vi "Inner Loop Control Select.vi"(8 "Inner Loop Gain Multiplier":dbl=1.0, 10 "Controller - User Input":T2={"Num Inner Loop"=[-11.0745, 19.702, -8.7598], "Den Inner Loop"=[1.0, -1.49756, 0.49756], "Inner Loop Gain"=1.0, "IMU_sample_rate"=0, "Num Outer Loop"=[0.1636, -0.16289, 0.0], "Den Outer Loop"=[1.0, -0.6326, 0.0], "Outer Loop Gain"=1.0, "Outer Loop sample rate"=20.0}, 11 "Controller Select":T1(ring)=enum."100hz/100hz" caption="Enum") -> (0 "Inner Loop Controller":T3, 4 "Outer Loop sample rate out":dbl)   [LabVIEW 2014]
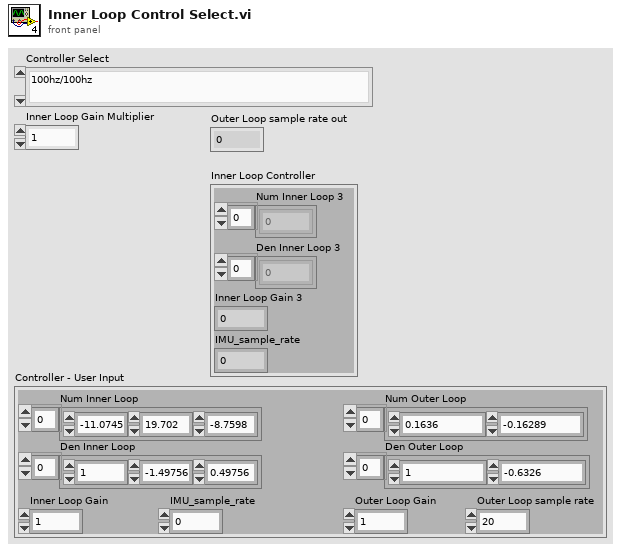
[diagram p1: front panel]
types:
  T1 = enum16{"100hz/50hz", "100hz/100hz", "200hz/200hz", "200hz/20hz", "User Defined"}
  T2 = cluster{"Num Inner Loop":dbl[], "Den Inner Loop":dbl[], "Inner Loop Gain":dbl, "IMU_sample_rate":i32, "Num Outer Loop":dbl[], "Den Outer Loop":dbl[], "Outer Loop Gain":dbl, "Outer Loop sample rate":dbl}
  T3 = cluster{"Num Inner Loop 3":dbl[], "Den Inner Loop 3":dbl[], "Inner Loop Gain 3":dbl, "IMU_sample_rate":i32}
  T4 = cluster{"Num Inner Loop":dbl[], "Den Inner Loop":dbl[], dbl, "IMU_sample_rate":i32}
  T5 = cluster{"Num Inner Loop 3":dbl[], "Den Inner Loop 3":dbl[], dbl, i32}
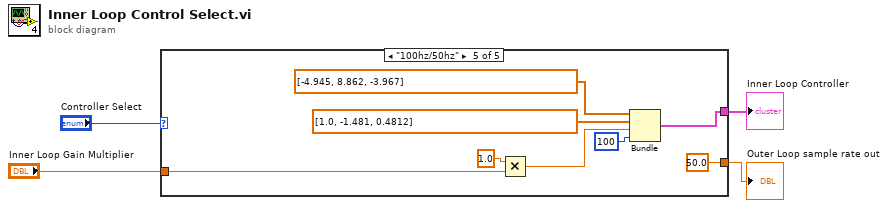
[diagram p0: block diagram]
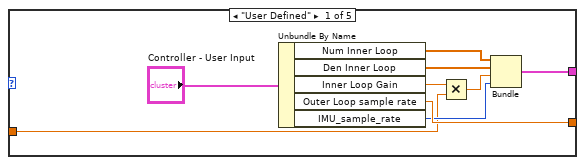
[diagram p2: hidden frame]
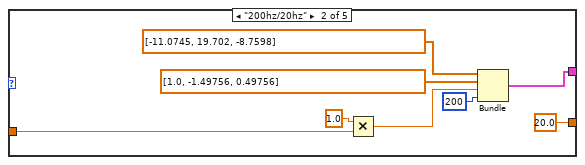
[diagram p3: hidden frame]
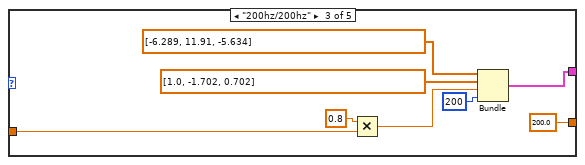
[diagram p4: hidden frame]
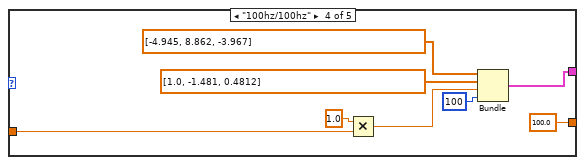
[diagram p5: hidden frame]
diagram:
  n1 = case shown="\"100hz/50hz\"" "Controller Select" {
    tunnel: [w13 20.0 ("Outer Loop sample rate") 200.0 ("Outer Loop sample rate") 100.0 ("Outer Loop sample rate") 50.0 ("Outer Loop sample rate")] -> w4
    tunnel: [w10 w18 w26 w34 w42] -> w3
    tunnel: "Inner Loop Gain Multiplier" -> [w7 w16 w24 w32 w38]
    frame "User Defined" {
      n2 = Unbundle By Name("Controller - User Input") -> ("Num Inner Loop"=w12:dbl[], "Den Inner Loop"=w11:dbl[], "Inner Loop Gain"=w5:dbl, "Outer Loop sample rate"=w13:dbl, "IMU_sample_rate"=w9:i32)
      n3 = Multiply(x=w5, y=w7) -> (x*y=w6:dbl)
      n4 = Bundle("Num Inner Loop"=w12, "Den Inner Loop"=w11, w6, "IMU_sample_rate"=w9) -> (w10:T4)  [unwired: 1 in]
    }
    frame "200hz/20hz" {
      n5 = Multiply(x=1.0 ("Inner Loop Gain 3"), y=w16) -> (x*y=w14:dbl)
      n6 = Bundle("Num Inner Loop 3"=dbl[] [-11.0745, 19.702, -8.7598], "Den Inner Loop 3"=dbl[] [1.0, -1.49756, 0.49756], w14, 200) -> (w18:T5)  [unwired: 1 in]
    }
    frame "200hz/200hz" {
      n7 = Multiply(x=0.8 ("Inner Loop Gain 3"), y=w24) -> (x*y=w22:dbl)
      n8 = Bundle("Num Inner Loop 3"=dbl[] [-6.289, 11.91, -5.634], "Den Inner Loop 3"=dbl[] [1.0, -1.702, 0.702], w22, 200) -> (w26:T5)  [unwired: 1 in]
    }
    frame "100hz/100hz" {
      n9 = Multiply(x=1.0 ("Inner Loop Gain 3"), y=w32) -> (x*y=w30:dbl)
      n10 = Bundle("Num Inner Loop 3"=dbl[] [-4.945, 8.862, -3.967], "Den Inner Loop 3"=dbl[] [1.0, -1.481, 0.4812], w30, 100) -> (w34:T5)  [unwired: 1 in]
    }
    frame "100hz/50hz" {
      n11 = Multiply(x=1.0 ("Inner Loop Gain 3"), y=w38) -> (x*y=w39:dbl)
      n12 = Bundle("Num Inner Loop 3"=dbl[] [-4.945, 8.862, -3.967], "Den Inner Loop 3"=dbl[] [1.0, -1.481, 0.4812], w39, 100) -> (w42:T5)  [unwired: 1 in]
    }
  }
  "Outer Loop sample rate out" <- w4
  "Inner Loop Controller" <- w3
